vi "AnimatorExample1.vi"() -> ()   [LabVIEW 2012]
uses:
  Control/AnimatorXControl.xctl
panel:
  out "String 2":string="Instructions:\n\nThe following animators implement a special right-click menu feature that allows you to configure each animator. Right-click one of the animators and choose Configuration... to display the configuration dialog box. You can specify options, such as animation images and frame rate, for the animator. Animators can work in two modes: Automatic and Use value. Under the Automatic mode, an animator automatically changes the current picture according to the frame rate that you specify. Under the Use value mode, an animator shows a picture according to the frame index value you input.\n\nAn animator has two properties--Frame rate and Reverse. Both properties take effect only when you set an animator to the Automatic mode. If an animator is in the Use value mode, you can set the current frame index by animator value.\n\nThe Animator Project example VI contains two animator XControls. This example sets both animators to the Automatic mode. Open the AnimatorProject.lvproj to view the structure of the XControls. Run this VI and try changing the frame rate of these animators. Then stop the VI."
  in  "Mixer speed":dbl(knob)=8.0 scale=0.0..25.0
  in  "AnimatorXControl-Mixer":u32(xcontrol)
  in  "Flow speed":dbl(knob)=5.0 scale=0.0..25.0
  in  "stop":bool
  in  "AnimatorXControl-Flow":u32(xcontrol)
  # "DSC Module Example Program\nAnimator XControl Example 1"
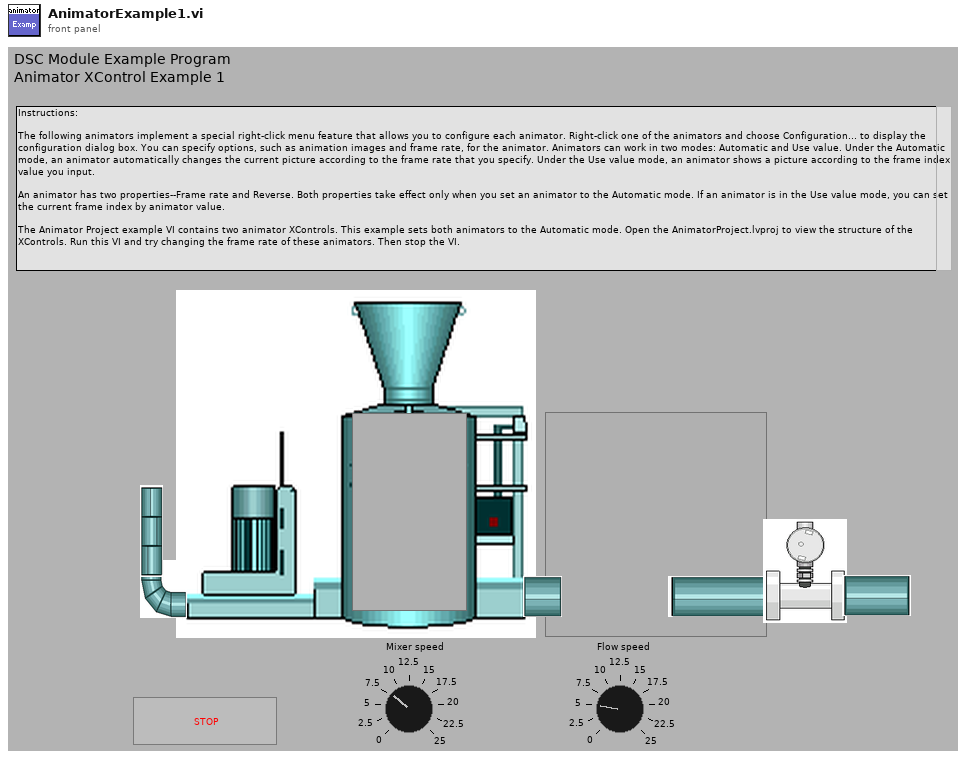
[diagram p1: front panel]
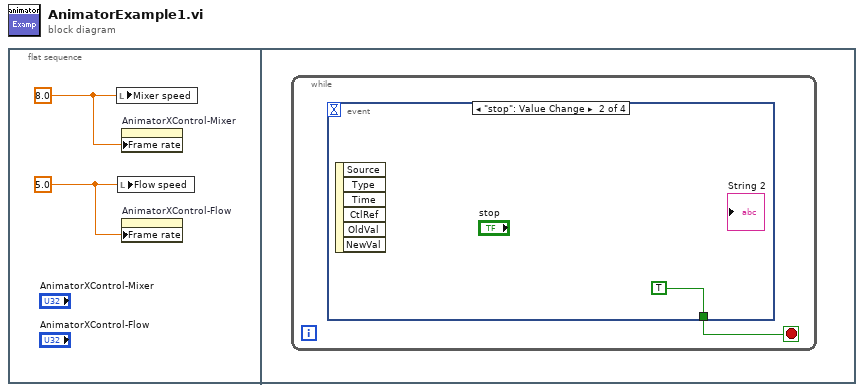
[diagram p0: block diagram]
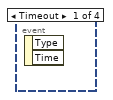
[diagram p2: hidden frame]
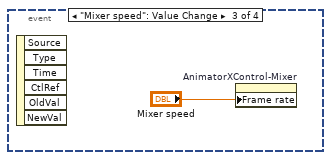
[diagram p3: hidden frame]
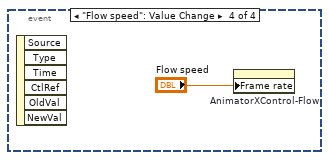
[diagram p4: hidden frame]
diagram:
  n1 = flat-sequence {
    frame #0 {
      w1 = 5.0 ("Speed 2")
      w2 = 8.0 ("Speed 1")
      n2 = local write "Mixer speed"(w2) -> ()
      n3 = local write "Flow speed"(w1) -> ()
      n4 = property on="AnimatorXControl-Mixer" class="AnimatorXControl (strict)"("Frame rate"=w2) -> ()  [unwired: 2 in, 2 out]
      n5 = property on="AnimatorXControl-Flow" class="AnimatorXControl (strict)"("Frame rate"=w1) -> ()  [unwired: 2 in, 2 out]
    }
    frame #1 {
      n6 = while {
        stop <- w3 stop-if-true
        n7 = event shown="[1] \"stop\": Value Change" {
          selector: _ -> [_ _ _ _]
          dyn-events: _ -> [_ _ _ _]
          timeout: _ -> [_ _ _ _]
          tunnel: [_ TRUE _ _] -> w3
          event Timeout {
            n8 = event-data() -> ()  [unwired: 1 in, 2 out]
          }
          event "stop": Value Change {
            n9 = event-data() -> ()  [unwired: 1 in, 6 out]
          }
          event "Mixer speed": Value Change {
            n10 = event-data() -> ()  [unwired: 1 in, 6 out]
            n11 = property on="AnimatorXControl-Mixer" class="AnimatorXControl (strict)"("Frame rate"="Mixer speed") -> ()  [unwired: 2 in, 2 out]
          }
          event "Flow speed": Value Change {
            n12 = event-data() -> ()  [unwired: 1 in, 6 out]
            n13 = property on="AnimatorXControl-Flow" class="AnimatorXControl (strict)"("Frame rate"="Flow speed") -> ()  [unwired: 2 in, 2 out]
          }
        }
      }
    }
  }
